vi "JKIFace.vi"() -> ()   [LabVIEW 2024]
uses:
  <vilib>/userDefined/High Color/IMAQdx.ctl
  <vilib>/vision/driver/NI_Vision_Acquisition_Software.lvlib
panel:
  in  "Tab Control 2":enum32{"Page 1", "Page 2", "Page 3"}(tab)
  in  "stop 2":bool
  out "Image 3":T1(plugin-control) caption="Image"
  in  "Plik wyjsciowy 2":path=path "f:/test.jpg"
  in  "Zapisz 2":bool
  in  "Password":string
  in  "User":string
  in  "Refresh Button":bool
  out "Answer":dbl
  in  "Numeric 2":dbl
  in  "Numeric":dbl
  in  "Stop Button":bool
  in  "Sciezka:  2":path=path "d:/img"
  out "Image 4":T1(plugin-control)
  in  "Kamera 2":T2
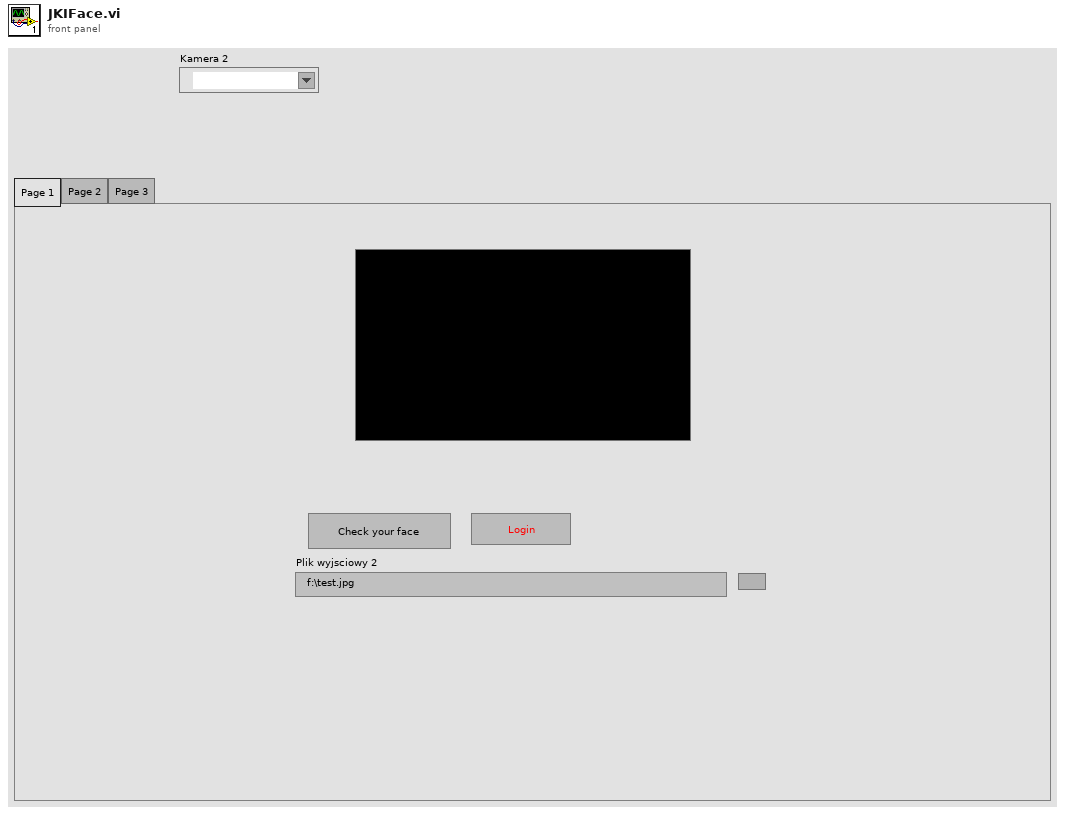
[diagram p1: front panel]
types:
  T1 = typedef "IMAQ Image.ctl" = refnum<image>
  T2 = typedef "IMAQdx.ctl" = refnum<k21>
  T3 = enum32{"Invalid", "Standard", "Closed", "Hidden", "Minimized", "Maximized"}
  T4 = enum32{"invalid app kind", "Development System", "Run Time System", "Student Edition", "Embedded LabVIEW", "Evaluation", "Custom"}
  T5 = cluster{"Core":cluster{"Current VI Reference":refnum<vi>, "Close Panel on Exit?":bool}, "Your Boolean data":bool, "Your string data":string, "Kamera 2":T2, "Sciezka:  2":path}
  T6 = cluster{"Current VI Reference":refnum<vi>, "Close Panel on Exit?":bool}
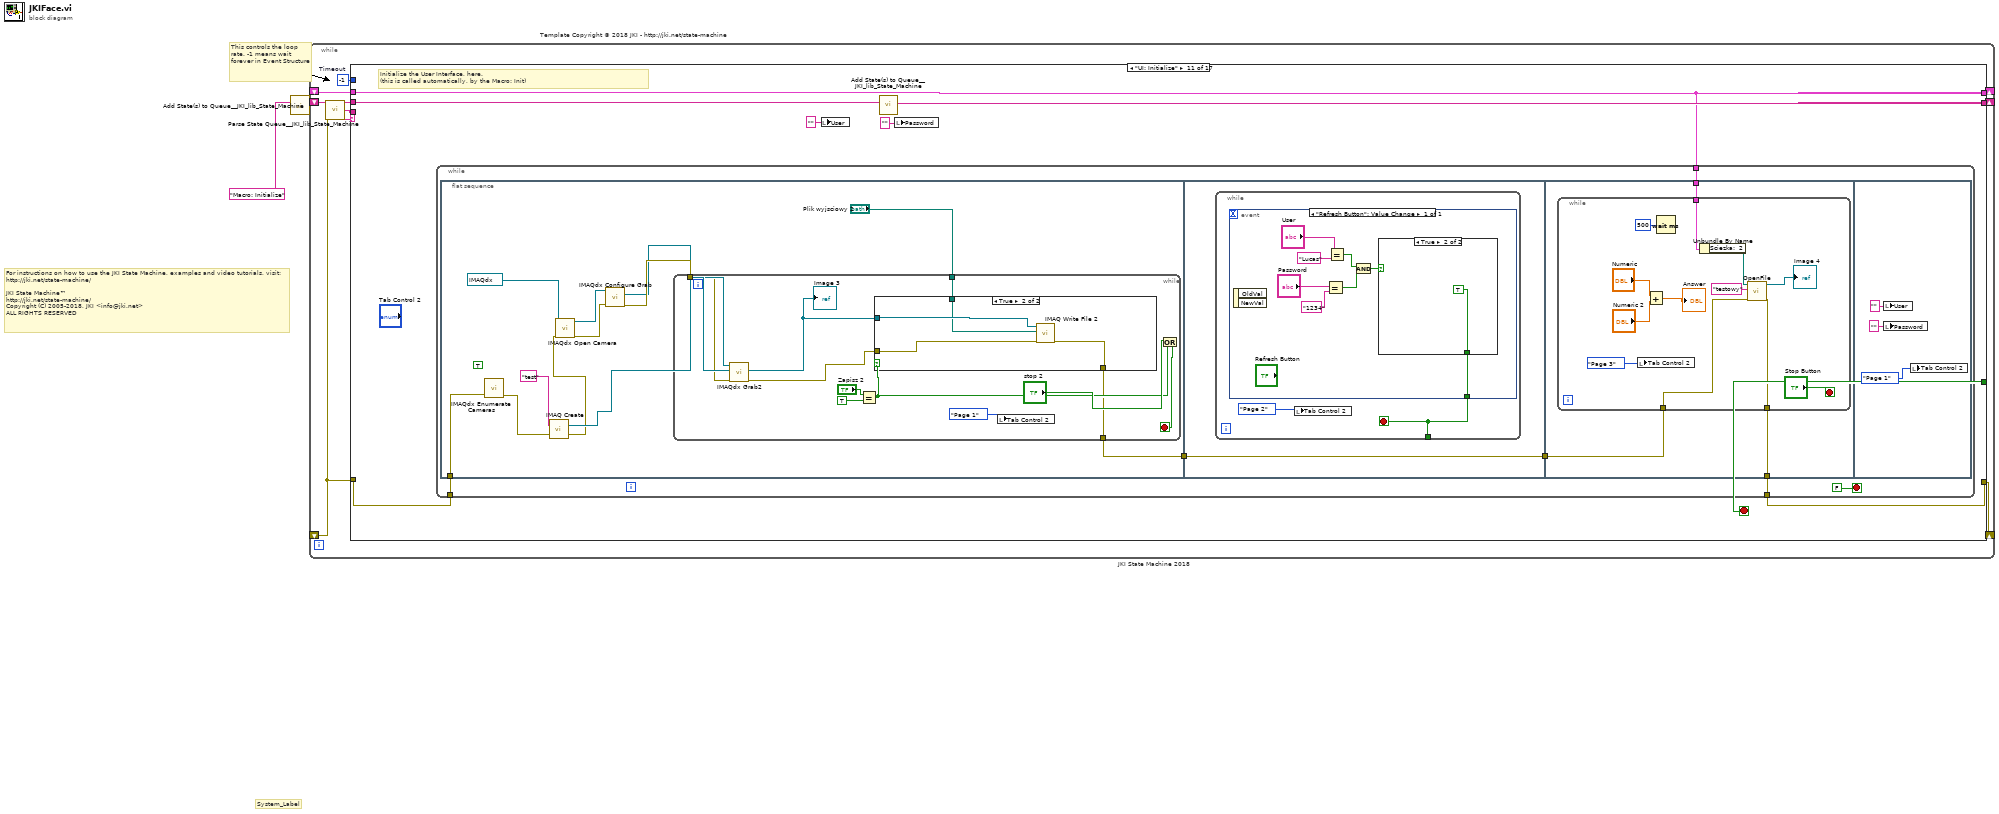
[diagram p0: block diagram]
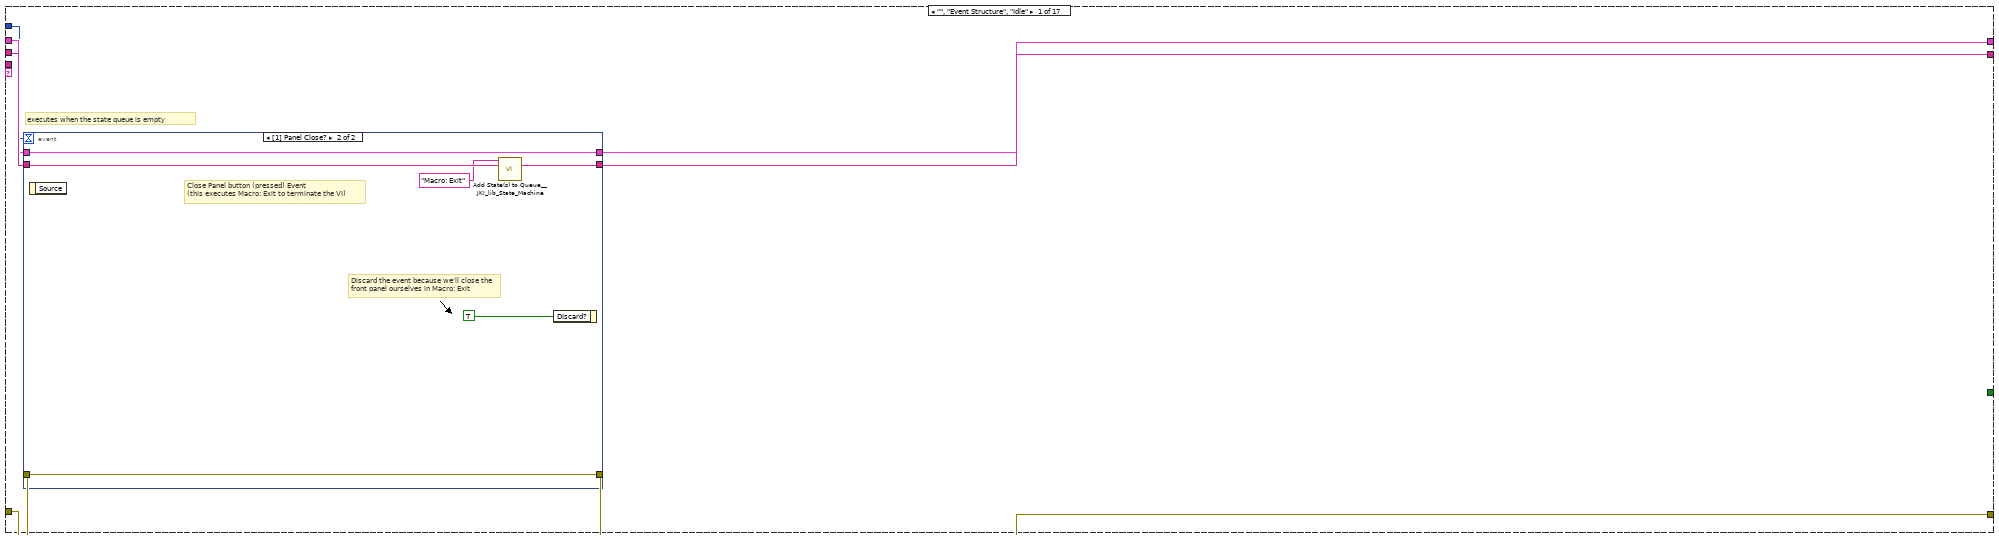
[diagram p2: hidden frame]
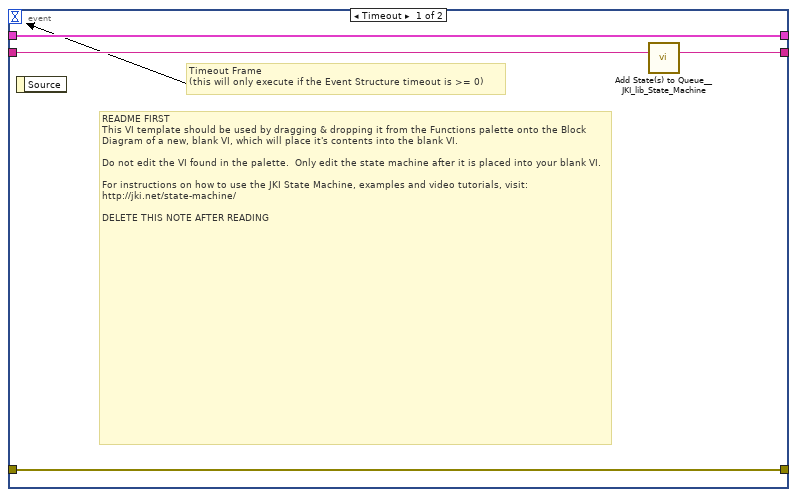
[diagram p3: hidden frame]
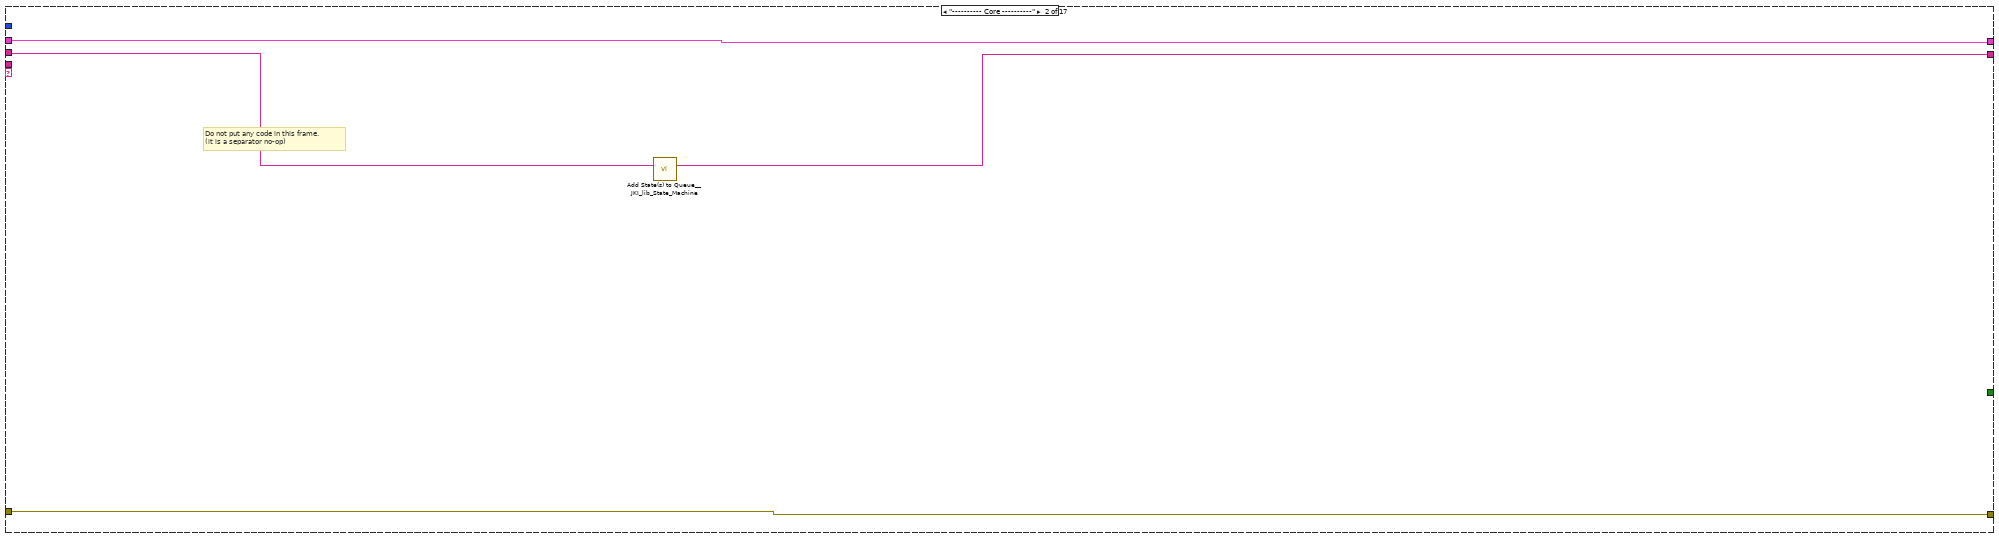
[diagram p4: hidden frame]
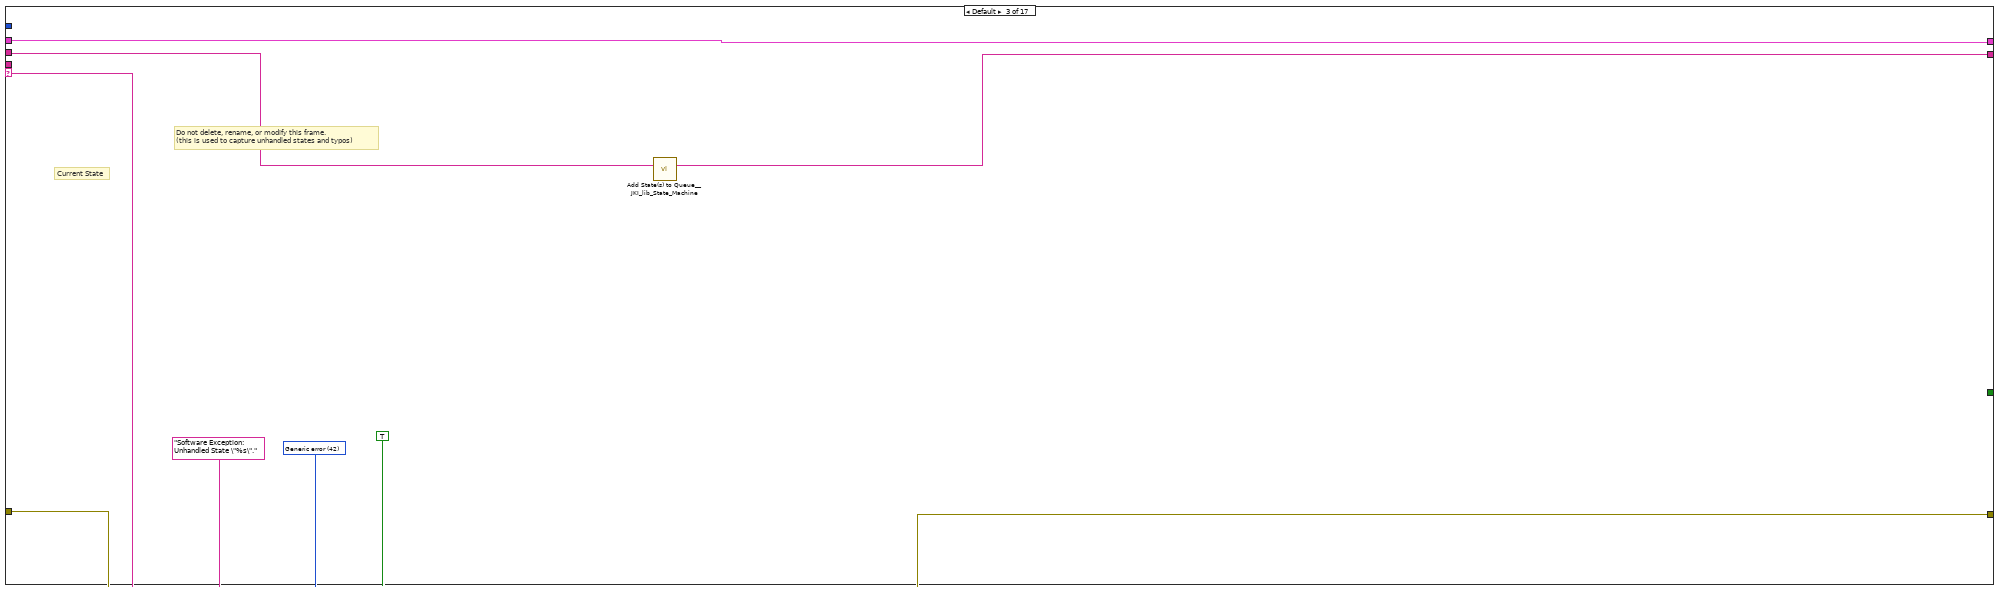
[diagram p5: hidden frame]
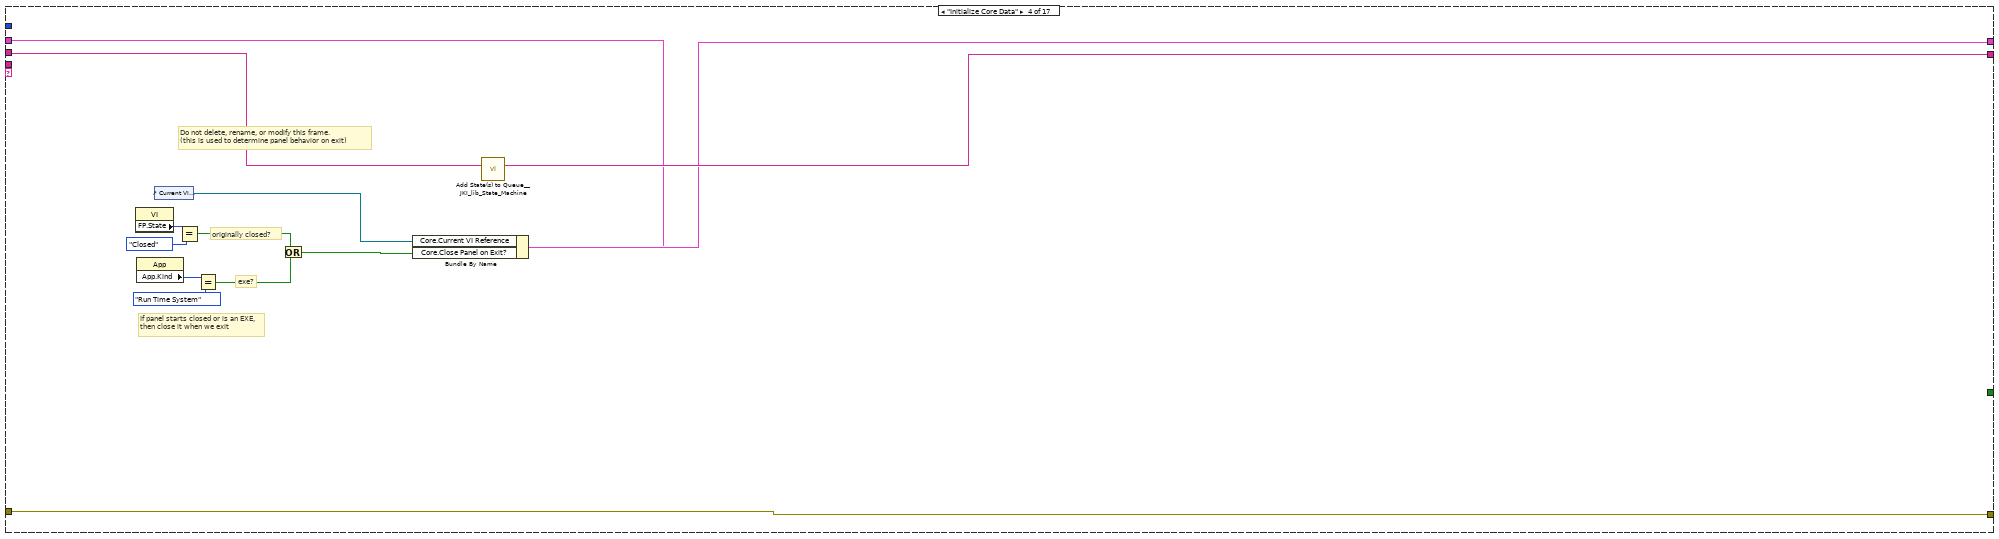
[diagram p6: hidden frame]
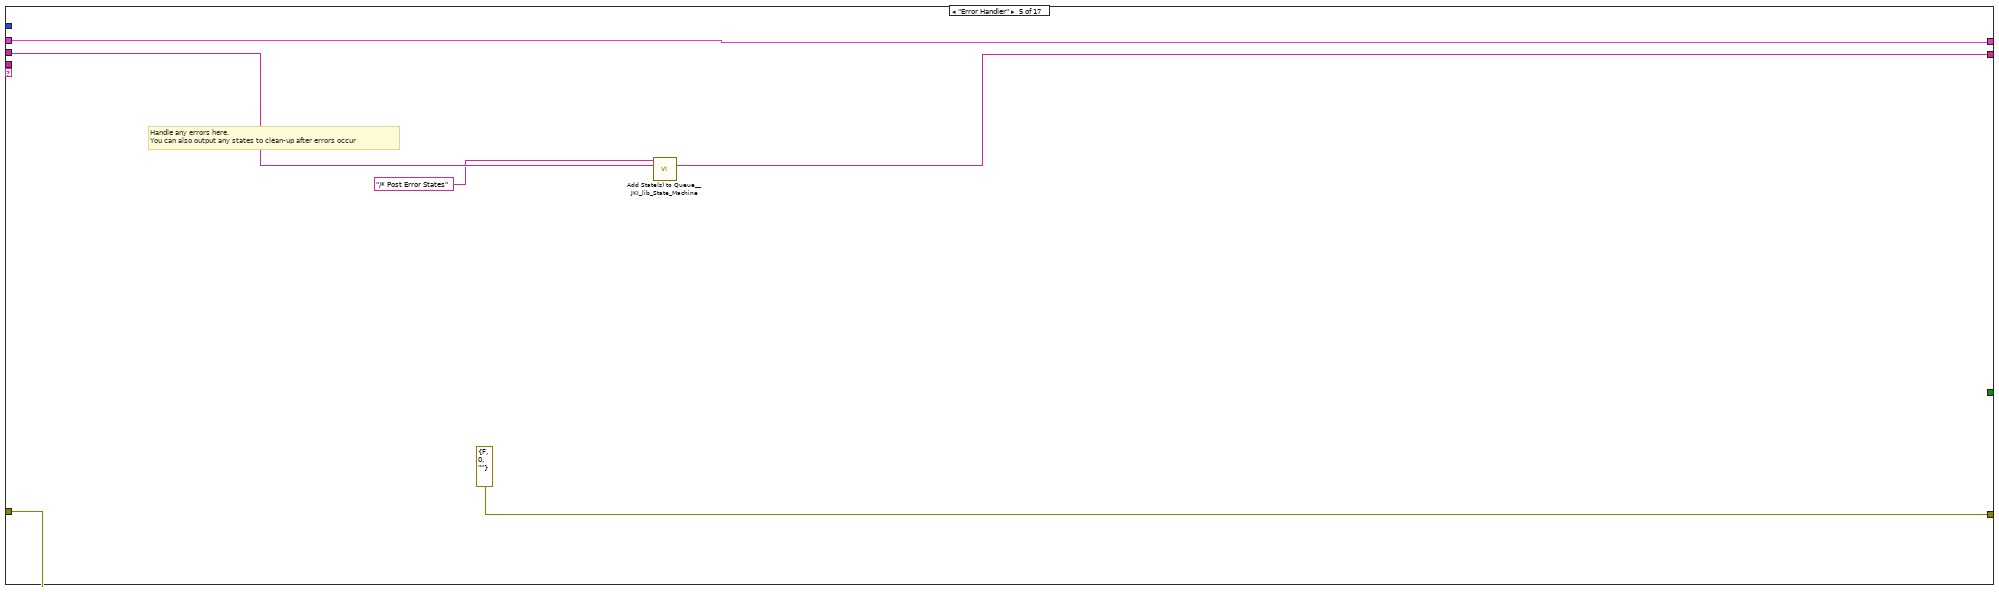
[diagram p7: hidden frame]
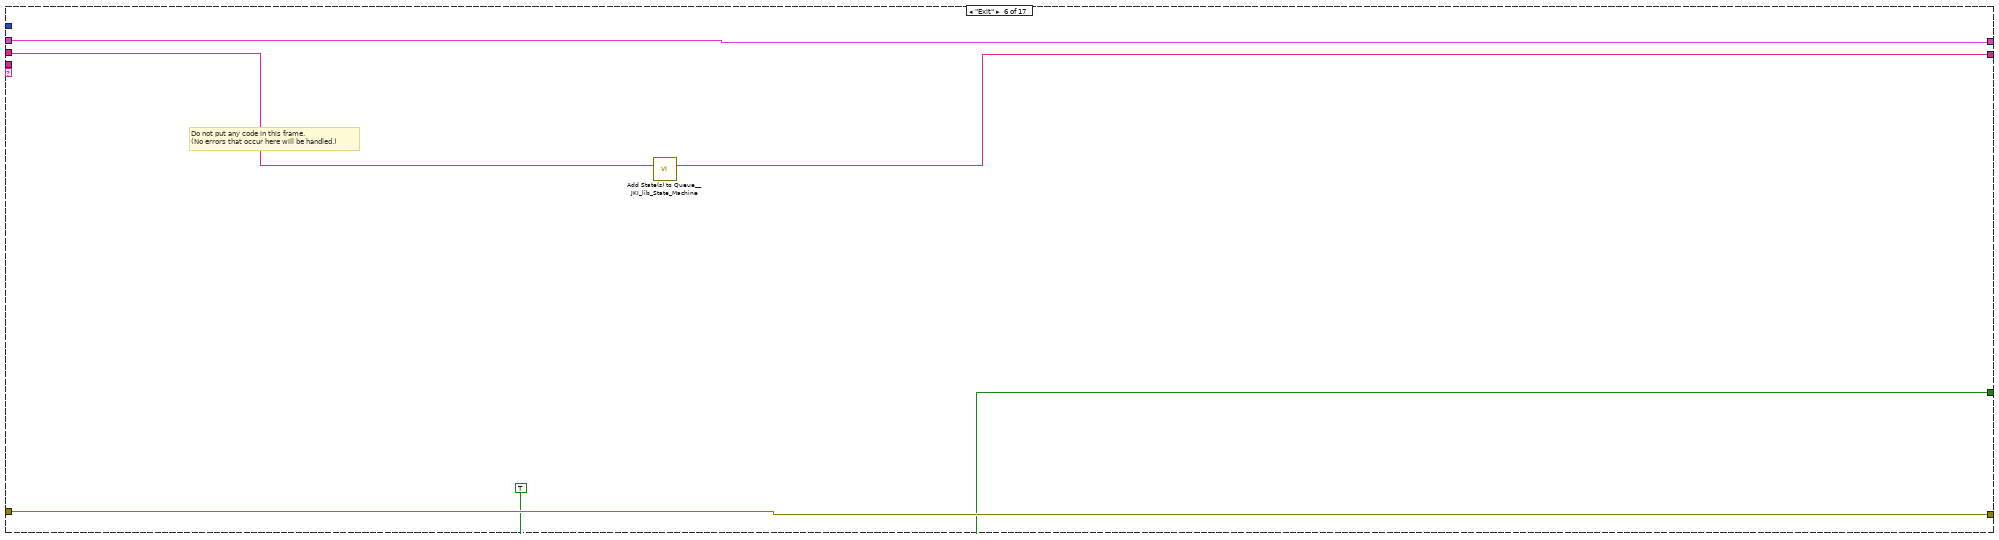
[diagram p8: hidden frame]
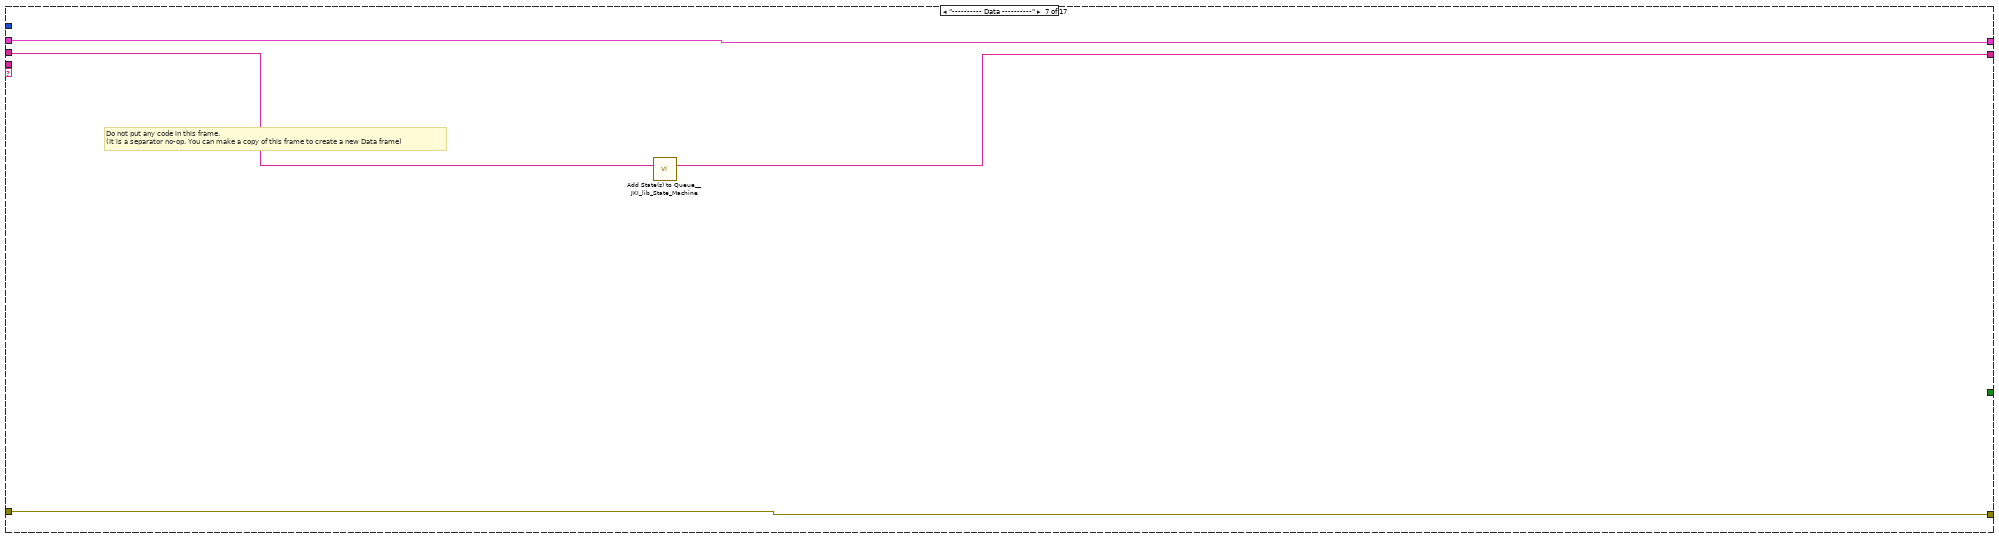
[diagram p9: hidden frame]
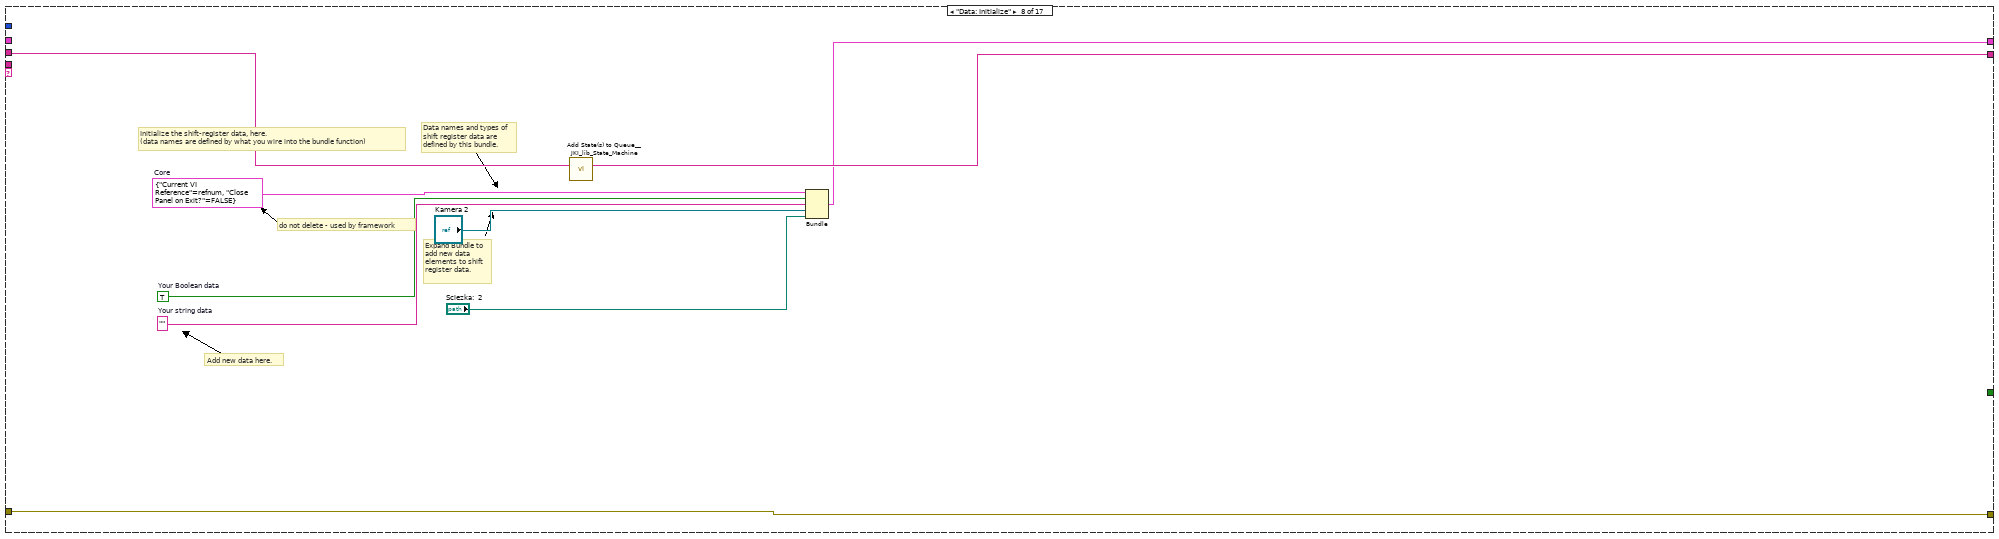
[diagram p10: hidden frame]
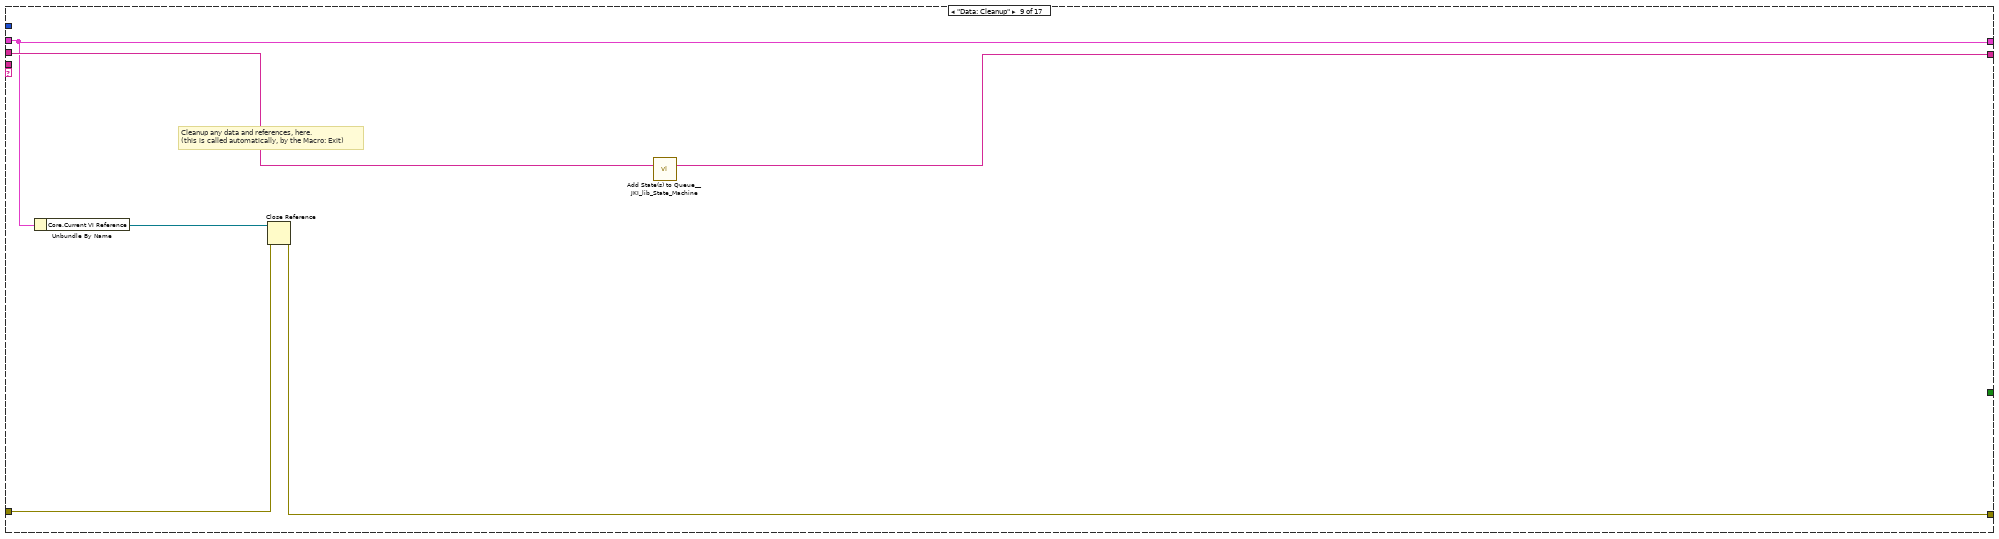
[diagram p11: hidden frame]
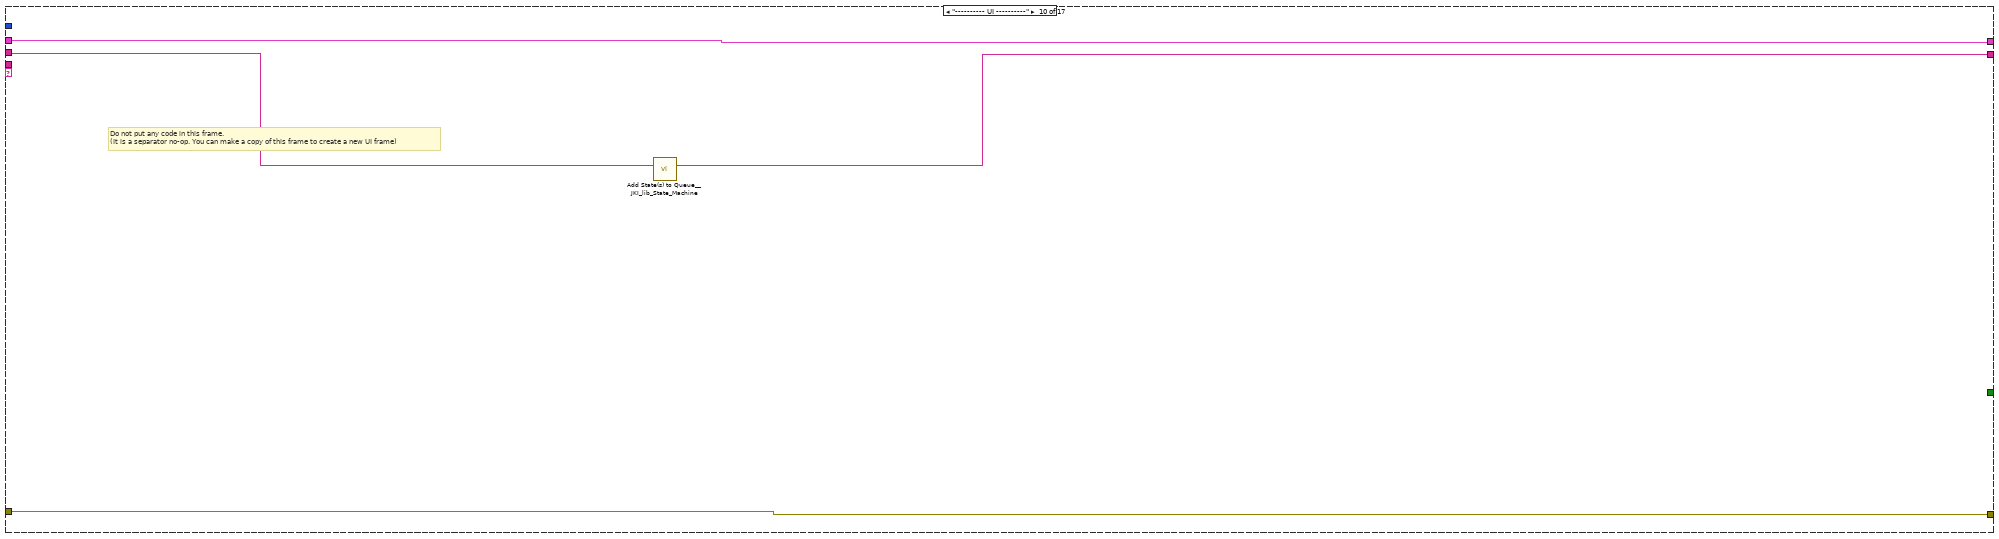
[diagram p12: hidden frame]
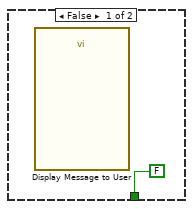
[diagram p14: hidden frame]
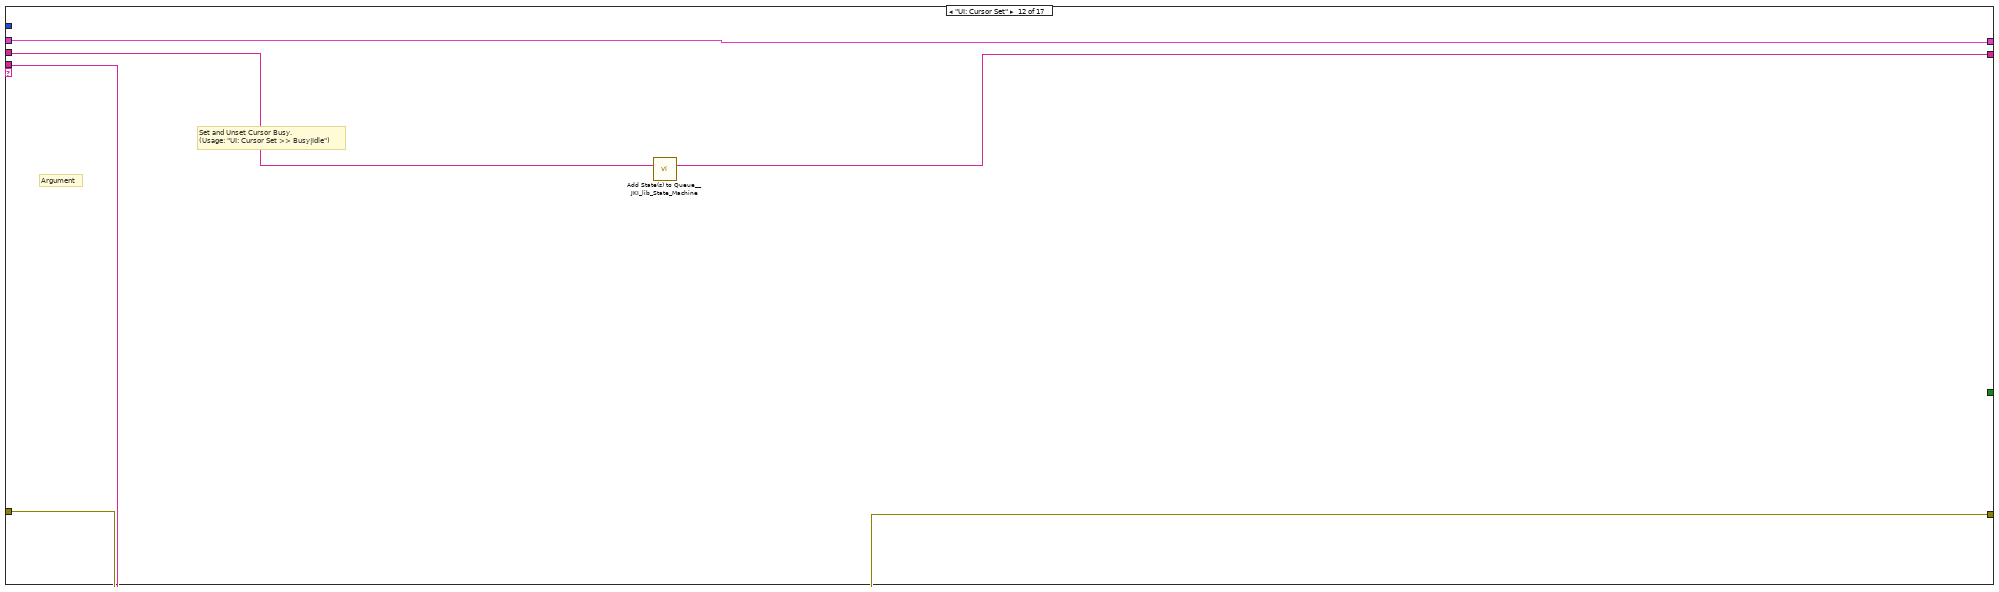
[diagram p15: hidden frame]
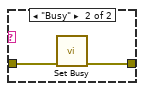
[diagram p16: hidden frame]
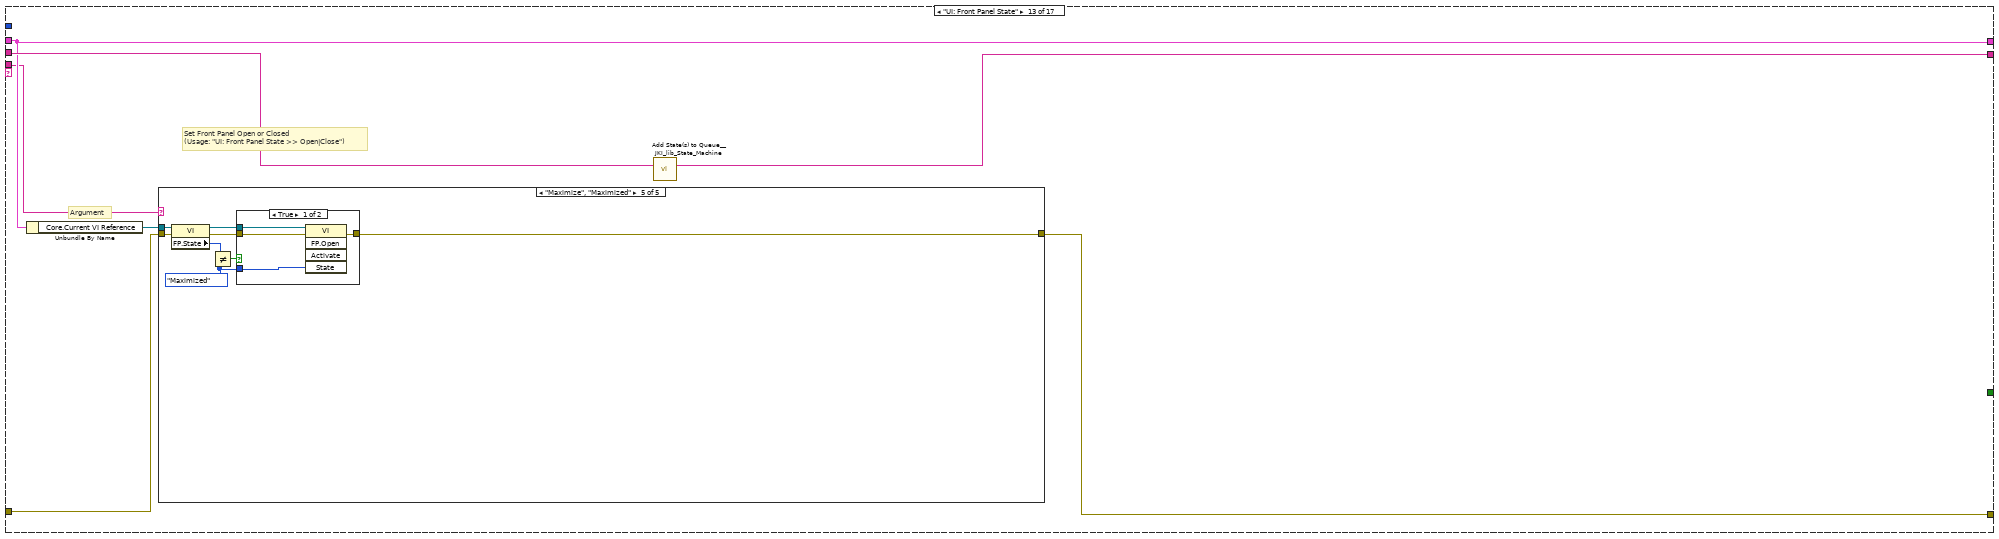
[diagram p17: hidden frame]
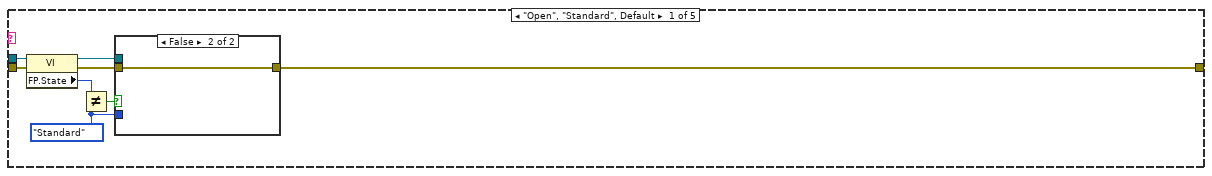
[diagram p18: hidden frame]
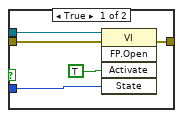
[diagram p19: hidden frame]
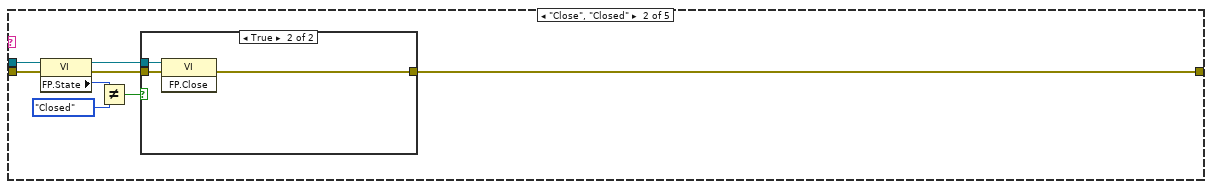
[diagram p20: hidden frame]
diagram:
  # "Template Copyright © 2018 JKI - http://jki.net/state-machine"
  # "For instructions on how to use the JKI State Machine, examples and video tutorials, visit:\nhttp://jki.net/state-machine/\n\nJKI State Machine™\nhttp://jki.net/state-machine/\nCopyright (C) 2005-2018, JKI <info@jki.net>\nALL RIGHTS RESERVED"
  # "This controls the loop rate. -1 means wait forever in Event Structure"
  # "System_Label"
  n1 = call <vilib>:"Add State(s) to Queue__JKI_lib_State_Machine.vi"("State(s) in (\"\")"="Macro: Initialize") -> ("States Out"=w2:string)  [unwired: 14 in]
  n2 = while "JKI State Machine 2018" {
    shift-right: [w6] -> _
    shift-left: _ -> [w5]
    shift-right: [w9] -> _
    shift-left: _ -> [w3]
    shift-right: [w8] -> _
    shift-left: w2 -> [w10]
    stop <- w7 stop-if-true
    w4 = -1  # Timeout
    n3 = call <vilib>:"Parse State Queue__JKI_lib_State_Machine.vi"("State Queue"=w10, "Error In (no error)"=w3) -> ("Remaining States"=w12:string, "Current State"=w13:string, "Arguments"=w11:string)  [unwired: 11 in]
    n4 = case shown="\"UI: Initialize\"" w13 {
      selector: w13 -> [_ _ w35 _ _ _ _ _ _ _ _ _ _ _ _ _ _]
      tunnel: w12 -> [w20 w34 w39 w58 w64 w69 w73 w82 w88 w92 w99 w172 w183 w252 w257 w267 w271]
      tunnel: w11 -> [_ _ _ _ _ _ _ _ _ _ _ w167 w177 _ _ _ _]
      tunnel: w5 -> [w18 w31 w37 w51 w61 w67 w70 _ w83 w89 w95 w170 w179 w249 w254 w264 w268]
      tunnel: [w17 w32 w41 w55 errorcluster {"status"=FALSE, "code"=0, "source"=""} ("error out") w66 w71 w79 w84 w90 w94 w168 w180 w250 w255 w265 w269] -> w9
      tunnel: w3 -> [w16 w32 w40 w55 w60 w66 w71 w79 w85 w90 w93 w169 w181 w250 w255 w265 w269]
      tunnel: [w19 w33 w38 w57 w63 w68 w72 w81 w87 w91 w98 w171 w182 w251 w256 w266 w270] -> w8
      tunnel: [_ _ _ _ _ TRUE _ _ _ _ _ _ _ _ _ _ _] -> w7
      tunnel: [w15 w31 w37 w56 w61 w67 w70 w80 w83 w89 w95 w170 w179 w249 w254 w264 w268] -> w6
      tunnel: w4 -> [w14 _ _ _ _ _ _ _ _ _ _ _ _ _ _ _ _]
      frame "", "Event Structure", "Idle" {
        # "executes when the state queue is empty"
        n5 = event shown="[1] Panel Close?" {
          selector: _ -> [_ _]
          dyn-events: _ -> [_ _]
          timeout: w14 -> [_ _]
          tunnel: w20 -> [w24 w30]
          tunnel: [w23 w29] -> w19
          tunnel: w18 -> [w21 w27]
          tunnel: [w22 w28] -> w17
          tunnel: w16 -> [w22 w28]
          tunnel: [w21 w27] -> w15
          event Timeout {
            # "README FIRST\nThis VI template should be used by dragging & dropping it from the Functions palette onto the Block Diagram of a new, blank VI, which will place it's contents into the blank VI.\n\nDo not edit the VI found in the palette.  Only edit the state machine after it is placed into your blank VI.\n\nFor instructions on how to use the JKI State Machine, examples and video tutorials, visit:\nhttp://jki.net/state-machine/\n\nDELETE THIS NOTE AFTER READING"
            # "Timeout Frame\n(this will only execute if the Event Structure timeout is >= 0)"
            n6 = event-data() -> ()  [unwired: 1 in, 1 out]
            n7 = call <vilib>:"Add State(s) to Queue__JKI_lib_State_Machine.vi"("State(s) in (\"\")"=w24) -> ("States Out"=w23:string)  [unwired: 14 in]
          }
          event Panel Close? {
            # "Discard the event because we'll close the front panel ourselves in Macro: Exit"
            # "Close Panel button (pressed) Event\n(this executes Macro: Exit to terminate the VI)"
            n8 = event-data() -> ()  [unwired: 1 in, 1 out]
            n9 = call <vilib>:"Add State(s) to Queue__JKI_lib_State_Machine.vi"("State(s) in Front (\"\")"="Macro: Exit", "State(s) in (\"\")"=w30) -> ("States Out"=w29:string)  [unwired: 13 in]
            n10 = event-data("Discard?"=TRUE) -> ()  [unwired: 1 in, 1 out]
          }
        }
      }
      frame "---------- Core ----------" {
        # "Do not put any code in this frame.\n(it is a separator no-op)"
        n11 = call <vilib>:"Add State(s) to Queue__JKI_lib_State_Machine.vi"("State(s) in (\"\")"=w34) -> ("States Out"=w33:string)  [unwired: 14 in]
      }
      frame Default {
        w44 = 42 items=["No error", "Argument error", "Memory is full", "Out of zone", "End of file", "File already open", "Generic file I/O error", "File not found", "File permission error", "Disk is full", "Duplicate path", "Too many files open", "System feature not enabled", "Resource file not found", "Cannot add resource", "Resource not found", "Image not found", "Image memory error", "Pen does not exist", "Config type invalid", "Config token not found", "Config parse error", "Config memory error", "Bad external code format", "Bad external code offset", "External code not present", "Null window", "Destroy window error", "Null menu", "Print aborted", "Bad print record", "Print driver error", "Windows error during printing", "Memory error during printing", "Print dialog error", "Generic print error", "Invalid device refnum", "Device not found", "Device parameter error", "Device unit error", "Cannot open device", "Device call aborted", "Generic error", "Cancelled by user", "Object ID too low", "Object ID too high", "Object not in heap", "Unknown heap", "Unknown object (invalid DefProc)", "Unknown object (DefProc not in table)", "Message out of range", "Invalid (null) method", "Unknown message", "Manager call not supported", "Bad address", "Network operation in progress", "Network operation timed out", "Connection is busy", "Network attribute not supported", "Network error", "Address in use", "System out of memory", "Connection aborted", "Connection refused", "Not connected", "Already connected", "Connection closed", "Initialization error (interapplication manager)", "Bad occurrence", "Wait on unbound occurrence handler", "Occurrence queue overflow", "Datalog type conflict", "Unused", "Unrecognized type (interapplication manager)", "Memory corrupt", "Failed to make temporary DLL", "Old CIN version", "Drag socket not found", "Failed to load drop-object", "Failed to register OLE object", "Failed to release OLE object", "Format specifier type mismatch", "Unknown format specifier", "Too few format specifiers", "Too many format specifiers", "Scan failed", "Newer CIN version", "Error converting to variant", "Runtime menu error", "Password tampered", "Variant attribute not found", "Incompatible variant data type", "Event data is not available", "Event Store is not present", "Occurrence is not found", "Event Queue is not created", "Event info is not available", "Refnum passed is NULL", "Error retrieving Class GUID", "Error retrieving CoClass GUID", "Error retrieving TypeLib GUID.", "Bad built application magic bytes.", "Specific driver is different from the specific driver associated with the Logical Name.", "There is no session opened to the class driver.", "Max Error", "MAX - Error with config objects", "MAX - Error loading configuration", "MAX - Group not supported"]
        # "Current State"
        # "Do not delete, rename, or modify this frame.\n(this is used to capture unhandled states and typos)"
        # "Handle mistyped state name (developer tool)"
        n12 = Format Into String(format string="Software Exception: Unhandled State \"%s\"." ("message"), error in=w40, w35) -> (resulting string=w43:string, error out=w42:errorcluster)  [unwired: 1 in]
        n13 = call <vilib>:"Error Cluster From Error Code.vi"("show call chain? (False)"=TRUE, "error in (no error)"=w42, "error message (\"\")"=w43, "error code (0)"=w44) -> ("error out"=w41:errorcluster)  [unwired: 5 in]
        n14 = call <vilib>:"Add State(s) to Queue__JKI_lib_State_Machine.vi"("State(s) in (\"\")"=w39) -> ("States Out"=w38:string)  [unwired: 14 in]
      }
      frame "Initialize Core Data" {
        # "Do not delete, rename, or modify this frame.\n(this is used to determine panel behavior on exit)"
        # "originally closed?"
        # "exe?"
        # "If panel starts closed or is an EXE, then close it when we exit"
        n15 = property class="VI"() -> ("FP.State"=w48:T3)  [unwired: 2 in, 2 out]
        n16 = property class="App"() -> ("App.Kind"=w54:T4)  [unwired: 2 in, 2 out]
        n17 = control-ref of="Current VI Reference"() -> (w49:refnum<vi>)
        n18 = Equal?(x=w48, y=T3."Closed" ("Front Panel Window:State")) -> (x = y?=w46:bool)
        n19 = Equal?(x=w54, y=T4."Run Time System" ("Application:Kind")) -> (x = y?=w52:bool)
        n20 = Or(x=w46, y=w52) -> (x .or. y?=w50:bool)
        n21 = Bundle By Name(cluster=w51, "Core.Current VI Reference"=w49, "Core.Close Panel on Exit?"=w50) -> (w56:T5)
        n22 = call <vilib>:"Add State(s) to Queue__JKI_lib_State_Machine.vi"("State(s) in (\"\")"=w58) -> ("States Out"=w57:string)  [unwired: 14 in]
      }
      frame "Error Handler" {
        # "Unhandled Error -- Display it"
        # "Handle any errors here.\nYou can also output any states to clean-up after errors occur"
        # "Clear error"
        n23 = call <vilib>:"General Error Handler.vi"("error in (no error)"=w60) -> ()  [unwired: 10 in, 5 out]
        n24 = call <vilib>:"Add State(s) to Queue__JKI_lib_State_Machine.vi"("State(s) in Front (\"\")"="/* Post Error States", "State(s) in (\"\")"=w64) -> ("States Out"=w63:string)  [unwired: 13 in]
      }
      frame "Exit" {
        # "Do not put any code in this frame.\n(No errors that occur here will be handled.)"
        n25 = call <vilib>:"Add State(s) to Queue__JKI_lib_State_Machine.vi"("State(s) in (\"\")"=w69) -> ("States Out"=w68:string)  [unwired: 14 in]
      }
      frame "---------- Data ----------" {
        # "Do not put any code in this frame.\n(It is a separator no-op. You can make a copy of this frame to create a new Data frame)"
        n26 = call <vilib>:"Add State(s) to Queue__JKI_lib_State_Machine.vi"("State(s) in (\"\")"=w73) -> ("States Out"=w72:string)  [unwired: 14 in]
      }
      frame "Data: Initialize" {
        w76 = T6 {"Current VI Reference"=refnum, "Close Panel on Exit?"=FALSE}  # Core
        w78 = TRUE  # Your Boolean data
        w77 = ""  # Your string data
        # "do not delete - used by framework"
        # "Expand Bundle to add new data elements to shift register data."
        # "Add new data here."
        # "Data names and types of shift register data are defined by this bundle."
        # "Initialize the shift-register data, here.\n(data names are defined by what you wire into the bundle function)"
        n27 = call <vilib>:"Add State(s) to Queue__JKI_lib_State_Machine.vi"("State(s) in (\"\")"=w82) -> ("States Out"=w81:string)  [unwired: 14 in]
        n28 = Bundle("Core"=w76, "Your Boolean data"=w78, "Your string data"=w77, "Kamera 2"="Kamera 2", "Sciezka:  2"="Sciezka:  2") -> (w80:T5)  [unwired: 1 in]
      }
      frame "Data: Cleanup" {
        # "Cleanup any data and references, here.\n(this is called automatically, by the Macro: Exit)"
        n29 = Unbundle By Name(w83) -> ("Core.Current VI Reference"=w86:refnum<vi>)
        n30 = Close Reference(reference=w86, error in (no error)=w85) -> (error out=w84:errorcluster)
        n31 = call <vilib>:"Add State(s) to Queue__JKI_lib_State_Machine.vi"("State(s) in (\"\")"=w88) -> ("States Out"=w87:string)  [unwired: 14 in]
      }
      frame "---------- UI ----------" {
        # "Do not put any code in this frame.\n(It is a separator no-op. You can make a copy of this frame to create a new UI frame)"
        n32 = call <vilib>:"Add State(s) to Queue__JKI_lib_State_Machine.vi"("State(s) in (\"\")"=w92) -> ("States Out"=w91:string)  [unwired: 14 in]
      }
      frame "UI: Initialize" {
        # "Initialize the User Interface, here.\n(this is called automatically, by the Macro: Init)"
        n33 = while {
          tunnel: w95 -> [w104]
          tunnel: [w103] -> w94
          tunnel: w93 -> [w102]
          stop <- FALSE stop-if-true
          n34 = flat-sequence {
            tunnel: w102 -> [w107]
            tunnel: [w106] -> w100
            tunnel: [w136] -> w101
            tunnel: w100 -> [w136]
            tunnel: w104 -> [w151]
            tunnel: [w150] -> w103
            tunnel: w101 -> [w149]
            frame #0 {
              (unwired) TRUE ("Connected Only? (Yes)")
              n35 = call <vilib>:"IMAQdx Enumerate Cameras.vi"("error in"=w107) -> ("error out"=w110:errorcluster)  [unwired: 9 in, 1 out]
              n36 = call "IMAQ Create"("Image Name"="test", "error in (no error)"=w110) -> ("New Image"=w112:T1, "error out"=w111:errorcluster)  [unwired: 2 in, 1 out]
              n37 = call <vilib>:"IMAQdx Open Camera.vi"("error in"=w111, "Session In"=T2 "cam0") -> ("error out"=w114:errorcluster, "Session Out"=w113:T2)  [unwired: 1 in, 7 out]
              n38 = call <vilib>:"IMAQdx Configure Grab.vi"("error in"=w114, "Session In"=w113) -> ("error out"=w117:errorcluster, "Session Out"=w116:T2)  [unwired: 8 in]
              n39 = while {
                tunnel: w112 -> [w127]
                tunnel: "Plik wyjsciowy 2" -> [w124]
                tunnel: w116 -> [w122]
                tunnel: w117 -> [w121]
                tunnel: [w118] -> w106
                stop <- w125 stop-if-true
                n40 = call <vilib>:"IMAQdx Grab2.vi"("error in"=w121, "Image In"=w127, "Session In"=w122) -> ("error out"=w128:errorcluster, "Image Out"=w123:T1)  [unwired: 5 in, 2 out]
                "Image 3" <- w123
                n41 = Equal?(x="Zapisz 2", y=TRUE) -> (x = y?=w120:bool)
                n42 = case shown="True" w120 {
                  tunnel: w128 -> [w131 w135]
                  tunnel: w123 -> [_ w134]
                  tunnel: w124 -> [_ w133]
                  tunnel: [w131 w132] -> w118
                  frame False {
                  }
                  frame True {
                    n43 = call-poly "IMAQ Write File 2"("error in (no error)"=w135, "File Path"=w133, "Image"=w134) -> ("error out"=w132:errorcluster)  [unwired: 2 in, 6 out]
                  }
                }
                n44 = local write "Tab Control 2"(enum32{"Page 1", "Page 2", "Page 3"}."Page 1" ("Tab Control")) -> ()
                n45 = Or(x="stop 2", y=w120) -> (x .or. y?=w125:bool)
              }
            }
            frame #1 {
              n46 = while {
                tunnel: [w138] -> _
                stop <- w138 stop-if-true
                n47 = event shown="[0] \"Refresh Button\": Value Change" {
                  selector: _ -> [_]
                  dyn-events: _ -> [_]
                  timeout: _ -> [_]
                  tunnel: [w139] -> w138
                  event "Refresh Button": Value Change {
                    n48 = event-data() -> ()  [unwired: 1 in, 2 out]
                    n49 = Equal?(x="Password", y="1234" ("x")) -> (x = y?=w141:bool)
                    n50 = Equal?(x="User", y="Lucas") -> (x = y?=w142:bool)
                    n51 = And(x=w142, y=w141) -> (x .and. y?=w140:bool)
                    n52 = case shown="True" w140 {
                      tunnel: [FALSE TRUE] -> w139
                      frame False {
                        n53 = call "Display Message to User"() -> ()  [unwired: 10 in, 2 out]
                      }
                      frame True {
                      }
                    }
                  }
                }
                n54 = local write "Tab Control 2"(enum32{"Page 1", "Page 2", "Page 3"}."Page 2" ("Tab Control")) -> ()
              }
            }
            frame #2 {
              n55 = while {
                tunnel: w151 -> [w157]
                tunnel: [w154] -> w150
                tunnel: w149 -> [w153]
                stop <- "Stop Button" stop-if-true
                n56 = local write "Tab Control 2"(enum32{"Page 1", "Page 2", "Page 3"}."Page 3" ("Tab Control")) -> ()
                n57 = Add(x="Numeric", y="Numeric 2") -> (x+y=→"Answer":dbl)
                n58 = Wait (ms)(milliseconds to wait=u32 500) -> ()  [unwired: 1 out]
                n59 = Unbundle By Name(w157) -> ("Sciezka:  2"=w156:path)
                n60 = call "OpenFile.vi"("error in (no error)"=w153, "Nazwa obrazu: 3"="testowy", "Sciezka:  2"=w156) -> ("error out"=w154:errorcluster, "Image 2"=→"Image 4":T1)  [unwired: 7 in]
              }
            }
            frame #3 {
              n61 = local write "User"("" ("User")) -> ()
              n62 = local write "Password"("" ("Password")) -> ()
              n63 = local write "Tab Control 2"(enum32{"Page 1", "Page 2", "Page 3"}."Page 1" ("Tab Control")) -> ()
            }
          }
        }
        n64 = local write "User"("" ("User")) -> ()
        n65 = call <vilib>:"Add State(s) to Queue__JKI_lib_State_Machine.vi"("State(s) in (\"\")"=w99) -> ("States Out"=w98:string)  [unwired: 14 in]
        n66 = local write "Password"("" ("Password")) -> ()
      }
      frame "UI: Cursor Set" {
        # "Argument"
        # "Set and Unset Cursor Busy.\n(Usage: \"UI: Cursor Set >> Busy|Idle\")"
        n67 = case shown="\"Idle\", Default" w167 {
          tunnel: w169 -> [w174 w176]
          tunnel: [w173 w175] -> w168
          frame "Idle", Default {
            n68 = call <vilib>:"Unset Busy.vi"("error in (no error)"=w174) -> ("error out"=w173:errorcluster)  [unwired: 10 in]
          }
          frame "Busy" {
            n69 = call <vilib>:"Set Busy.vi"("error in (no error)"=w176) -> ("error out"=w175:errorcluster)  [unwired: 9 in, 1 out]
          }
        }
        n70 = call <vilib>:"Add State(s) to Queue__JKI_lib_State_Machine.vi"("State(s) in (\"\")"=w172) -> ("States Out"=w171:string)  [unwired: 14 in]
      }
      frame "UI: Front Panel State" {
        # "Argument"
        # "Set Front Panel Open or Closed\n(Usage: \"UI: Front Panel State >> Open|Close\")"
        n71 = Unbundle By Name(w179) -> ("Core.Current VI Reference"=w178:refnum<vi>)
        n72 = case shown="\"Maximize\", \"Maximized\"" w177 {
          tunnel: w181 -> [w189 w204 w215 w228 w241]
          tunnel: [w191 w205 w217 w230 w243] -> w180
          tunnel: w178 -> [w190 w202 w216 w229 w242]
          frame "Open", "Standard", Default {
            w184 = T3."Standard" ("State")
            n73 = property class="VI"(reference=w190, error in=w189) -> (reference out=w187:refnum<vi>, error out=w188:errorcluster, "FP.State"=w186:T3)
            n74 = Not Equal?(x=w186, y=w184) -> (x != y?=w185:bool)
            n75 = case shown="False" w185 {
              tunnel: [w195 w197] -> w191
              tunnel: w188 -> [w194 w197]
              tunnel: w187 -> [w193 _]
              tunnel: w184 -> [w192 _]
              frame True {
                n76 = invoke class="VI" method="FP.Open"(reference=w193, error in=w194, "Activate"=TRUE, "State"=w192) -> (error out=w195:errorcluster)  [unwired: 1 in, 4 out]
              }
              frame False {
              }
            }
          }
          frame "Close", "Closed" {
            n77 = property class="VI"(reference=w202, error in=w204) -> (reference out=w201:refnum<vi>, error out=w203:errorcluster, "FP.State"=w199:T3)
            n78 = Not Equal?(x=w199, y=T3."Closed" ("Front Panel Window:State")) -> (x != y?=w198:bool)
            n79 = case shown="True" w198 {
              tunnel: [w206 w209] -> w205
              tunnel: w203 -> [w206 w208]
              tunnel: w201 -> [_ w207]
              frame False {
              }
              frame True {
                n80 = invoke class="VI" method="FP.Close"(reference=w207, error in=w208) -> (error out=w209:errorcluster)  [unwired: 1 in, 2 out]
              }
            }
          }
          frame "Hidden", "Hide" {
            w210 = T3."Hidden" ("State")
            n81 = property class="VI"(reference=w216, error in=w215) -> (reference out=w213:refnum<vi>, error out=w214:errorcluster, "FP.State"=w212:T3)
            n82 = Not Equal?(x=w212, y=w210) -> (x != y?=w211:bool)
            n83 = case shown="True" w211 {
              tunnel: [w221 w222] -> w217
              tunnel: w214 -> [w220 w222]
              tunnel: w213 -> [w219 _]
              tunnel: w210 -> [w218 _]
              frame True {
                n84 = invoke class="VI" method="FP.Open"(reference=w219, error in=w220, "State"=w218) -> (error out=w221:errorcluster)  [unwired: 2 in, 4 out]
              }
              frame False {
              }
            }
          }
          frame "Minimize", "Minimized" {
            w223 = T3."Minimized" ("State")
            n85 = property class="VI"(reference=w229, error in=w228) -> (reference out=w226:refnum<vi>, error out=w227:errorcluster, "FP.State"=w225:T3)
            n86 = Not Equal?(x=w225, y=w223) -> (x != y?=w224:bool)
            n87 = case shown="True" w224 {
              tunnel: [w234 w235] -> w230
              tunnel: w227 -> [w233 w235]
              tunnel: w226 -> [w232 _]
              tunnel: w223 -> [w231 _]
              frame True {
                n88 = invoke class="VI" method="FP.Open"(reference=w232, error in=w233, "State"=w231) -> (error out=w234:errorcluster)  [unwired: 2 in, 4 out]
              }
              frame False {
              }
            }
          }
          frame "Maximize", "Maximized" {
            w236 = T3."Maximized" ("State")
            n89 = property class="VI"(reference=w242, error in=w241) -> (reference out=w239:refnum<vi>, error out=w240:errorcluster, "FP.State"=w238:T3)
            n90 = Not Equal?(x=w238, y=w236) -> (x != y?=w237:bool)
            n91 = case shown="True" w237 {
              tunnel: [w247 w248] -> w243
              tunnel: w240 -> [w246 w248]
              tunnel: w239 -> [w245 _]
              tunnel: w236 -> [w244 _]
              frame True {
                n92 = invoke class="VI" method="FP.Open"(reference=w245, error in=w246, "State"=w244) -> (error out=w247:errorcluster)  [unwired: 2 in, 4 out]
              }
              frame False {
              }
            }
          }
        }
        n93 = call <vilib>:"Add State(s) to Queue__JKI_lib_State_Machine.vi"("State(s) in (\"\")"=w183) -> ("States Out"=w182:string)  [unwired: 14 in]
      }
      frame "---------- Macro ----------" {
        # "Do not put any code in this frame.\n(It is a separator no-op. You can make a copy of this frame to create a new Macro frame)"
        n94 = call <vilib>:"Add State(s) to Queue__JKI_lib_State_Machine.vi"("State(s) in (\"\")"=w252) -> ("States Out"=w251:string)  [unwired: 14 in]
      }
      frame "Macro: Initialize" {
        # "Initialization Macro\n(This is called once, when the VI starts)"
        n95 = call <vilib>:"Add State(s) to Queue__JKI_lib_State_Machine.vi"("State(s) in Front (\"\")"="Data: Initialize\nInitialize Core Data\nUI: Initialize\nUI: Front Panel State >> Open\n \n\n", "State(s) in (\"\")"=w257) -> ("States Out"=w256:string)  [unwired: 13 in]
      }
      frame "Macro: Exit" {
        # "Exit Macro\n(This is called once, when the VI exits)"
        n96 = Unbundle By Name(w264) -> ("Core.Close Panel on Exit?"=w263:bool)
        n97 = Select(t="UI: Front Panel State >> Close", s=w263, f="") -> (s? t:f=w260:string)
        n98 = call <vilib>:"Add State(s) to Queue__JKI_lib_State_Machine.vi"("State(s) in (\"\")"=w260, "State(s) at Back (\"\")"="Data: Cleanup\nExit") -> ("States Out"=w258:string)  [unwired: 13 in]
        n99 = call <vilib>:"Add State(s) to Queue__JKI_lib_State_Machine.vi"("State(s) in Front (\"\")"=w258, "State(s) in (\"\")"=w267) -> ("States Out"=w266:string)  [unwired: 13 in]
      }
      frame "---------- Biometric Login ----------" {
        # "Template Separator\n(You can make a copy of, or modify, this frame)"
        n100 = call <vilib>:"Add State(s) to Queue__JKI_lib_State_Machine.vi"("State(s) in (\"\")"=w271) -> ("States Out"=w270:string)  [unwired: 14 in]
      }
    }
  }
